vi "InitModuleManager.vi"(8 "error in (no error)":errorcluster, 10 "mmanager":path, 11 "SensorInfos":T6) -> (0 "error out (no error)":errorcluster, 3 "Sensor Engine Datas":T1[](array[typedef]) {"MM Frames"."payload" format="%x"; "MM Frames"."timestamp" format="%<%.7X\n%x>T"; "MM Frames"."type" items=["FlexRay Data"=32, "FlexRay Null"=33, "FlexRay Symbol"=34, "Log Trigger"=225, "Start Trigger"=226]; "MM Frames"."cycle count" max=63 step=1})   [LabVIEW 2023, in "MM.lvlib"]
uses:
  MM.lvlib
  Shared/SensorInfos.ctl
  Shared/SensorInfo.ctl
  Shared/Sensor Name.ctl
  Shared/Protocol.ctl
  MM Data.ctl
  MM Objects.ctl
  MM Object.ctl
  Sensor Engine Data.ctl
  <vilib>/xnet/xnet.llb/XNET Frame FlexRay.ctl
  <vilib>/xnet/xnet.llb/XNET Frame Type FlexRay.ctl
  <vilib>/xnet/xnet.llb/XNET String To IO Name (Signal).vi
  <vilib>/xnet/xnet.llb/XNET Create Session (Conversion).vi
  <resource>/objmgr/xnet.rc
  Shared/Vires VTD Shared.lvlib
  Engine/Vires VTD Engine.lvlib
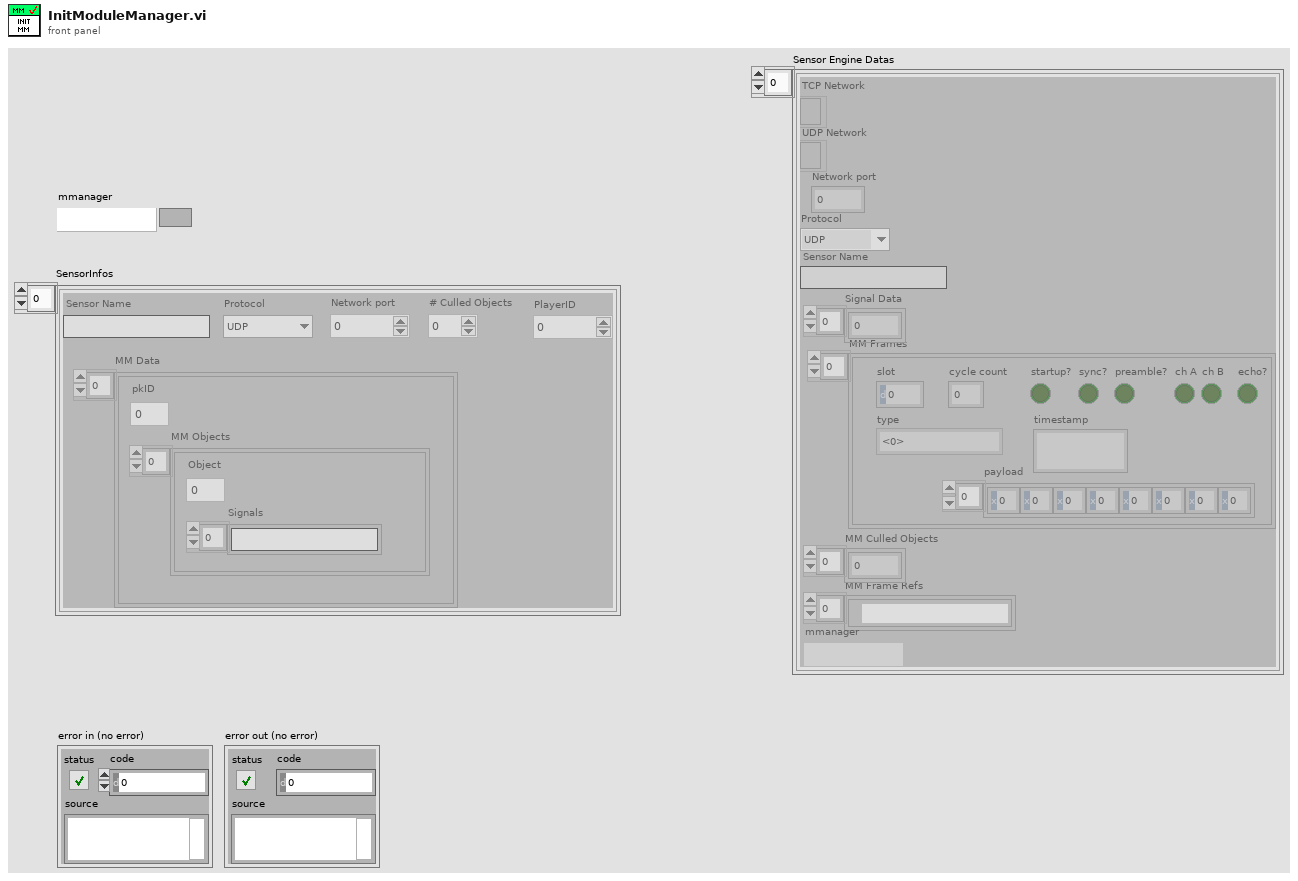
[diagram p1: front panel]
types:
  T1 = typedef "MM.lvlib/Sensor Engine Data.ctl" = cluster{"TCP Network":refnum<k5>, "UDP Network":refnum<k16>, "Network port":i32, "Protocol":T2, "Sensor Name":T3, "Signal Data":dbl[], "MM Frames":T4[], "MM Culled Objects":i32[], "MM Frame Refs":refnum<k21>[], "mmanager":path}
  T2 = typedef "Vires VTD Shared.lvlib/Protocol.ctl" = enum16{"UDP", "TCP"}
  T3 = typedef "Vires VTD Shared.lvlib/Sensor Name.ctl" = string
  T4 = typedef "XNET Frame FlexRay.ctl" = cluster{"timestamp":timestamp, "payload":u8[], "slot":u16, "type":T5, "cycle count":u8, "startup?":bool, "sync?":bool, "preamble?":bool, "ch A":bool, "ch B":bool, "echo?":bool}
  T5 = typedef "XNET Frame Type FlexRay.ctl" = u8
  T6 = typedef "Vires VTD Shared.lvlib/SensorInfos.ctl" = T7[]
  T7 = typedef "Vires VTD Shared.lvlib/SensorInfo.ctl" = cluster{"Sensor Name":T3, "Protocol":T2, "Network port":i32, "# Culled Objects":i32, "PlayerID":u8, "MM Data":T8}
  T8 = typedef "Vires VTD Shared.lvlib/MM Data.ctl" = T9[]
  T9 = typedef "MM.lvlib/MM Objects.ctl" = cluster{"pkID":i32, "MM Objects":T10[]}
  T10 = typedef "MM.lvlib/MM Object.ctl" = cluster{"Object":i32, "Signals":string[]}
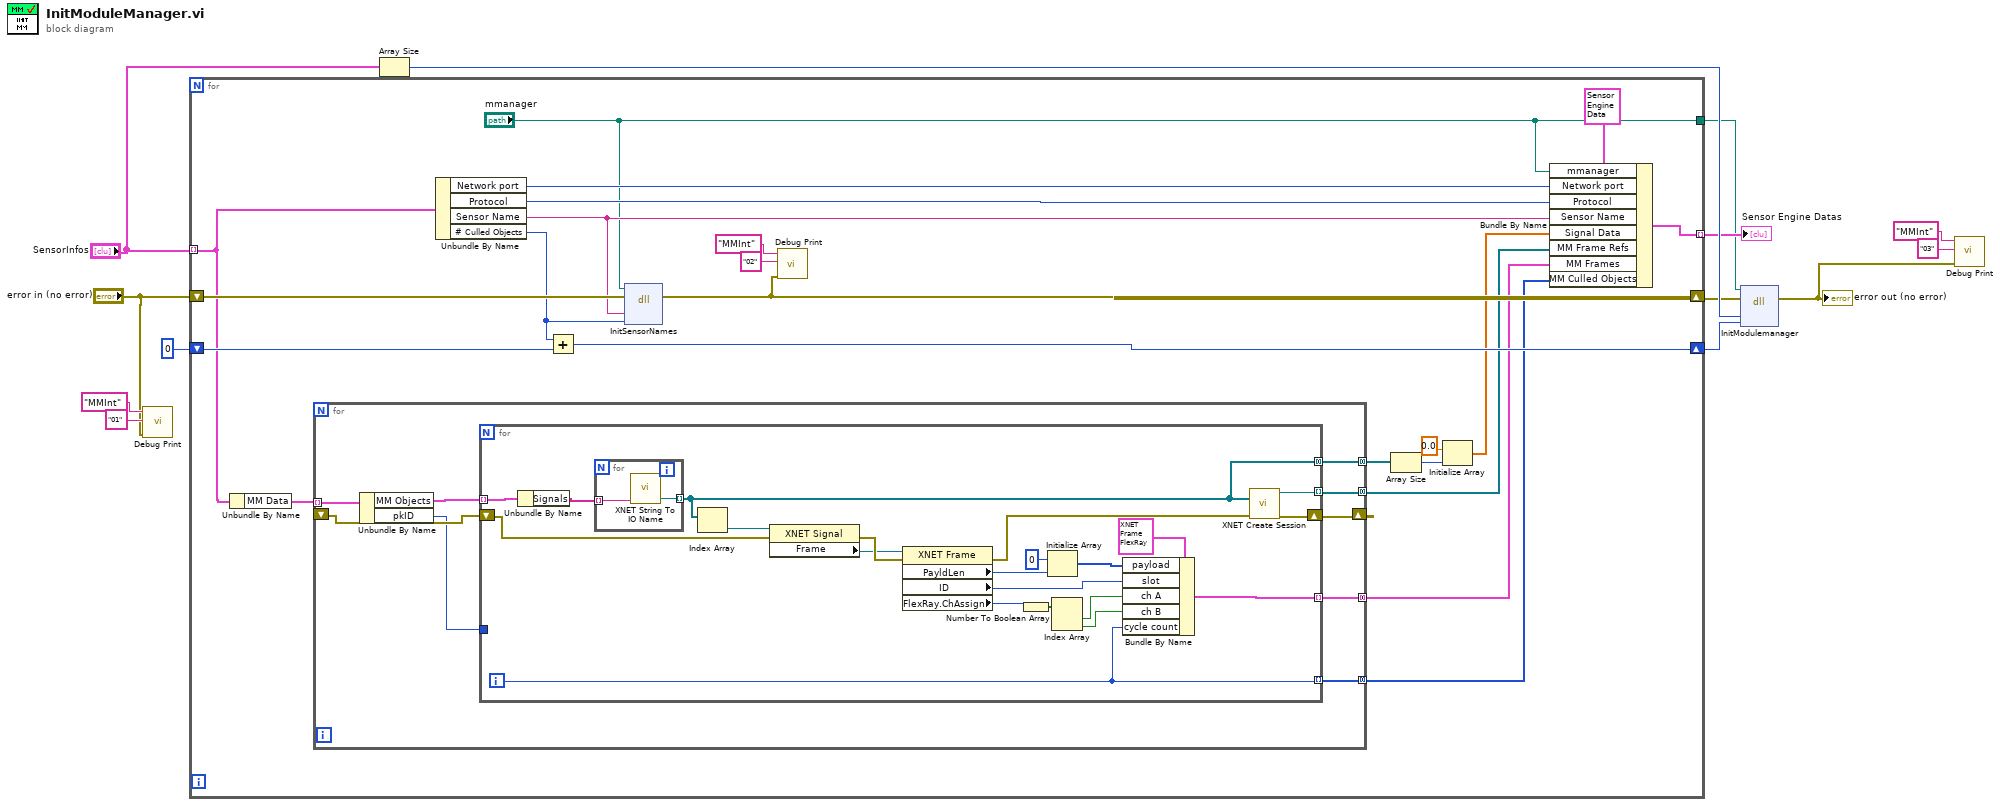
[diagram p0: block diagram]
diagram:
  n1 = call "Debug Print.vi"("error out"="error in (no error)", "Index"="01", "Module"="MMInt") -> ()  [unwired: 9 in]
  n2 = for {
    tunnel: "SensorInfos" -> [w31] mode=indexing
    shift-right: [w35] -> w11
    shift-left: 0 -> [w34]
    shift-right: [w14] -> w10
    shift-left: "error in (no error)" -> [w33]
    tunnel: [w19] -> w8 mode=indexing
    tunnel: ["mmanager"] -> w7
    n3 = Unbundle By Name(w31) -> ("MM Data"=w30:T8)
    n4 = for {
      shift-right: [w44] -> _
      shift-left: _ -> [w43]
      tunnel: [w42] -> w22 mode=concatenating
      tunnel: [w41] -> w21 mode=concatenating
      tunnel: w30 -> [w40] mode=indexing
      tunnel: [w37] -> w20 mode=concatenating
      tunnel: [w36] -> w18 mode=concatenating
      n5 = Unbundle By Name(w40) -> ("MM Objects"=w39:T10[], "pkID"=w38:i32)
      n6 = for {
        tunnel: [w52] -> w41 mode=indexing
        tunnel: [w48] -> w42 mode=indexing
        shift-right: [w50] -> w44
        shift-left: w43 -> [w49]
        tunnel: w39 -> [w47] mode=indexing
        tunnel: w38 -> [_]
        tunnel: [w46] -> w37 mode=indexing
        tunnel: [w45] -> w36 mode=concatenating
        i -> [w46]
        n7 = Unbundle By Name(w47) -> ("Signals"=w65:string[])
        n8 = for {
          tunnel: w65 -> [w67] mode=indexing
          tunnel: [w66] -> w45 mode=indexing
          n9 = call-poly <vilib>:"XNET String To IO Name.vi"("string"=w67) -> ("XNET Signal"=w66:refnum<k21>)  [unwired: 4 out]
        }
        n10 = Index Array(array=w45) -> (element=w53:refnum<k21>)  [unwired: 1 in]
        n11 = property class="XNET Signal"(reference=w53, error in=w49) -> (error out=w64:errorcluster, "Frame"=w63:refnum<k21>)  [unwired: 1 out]
        n12 = property class="XNET Frame"(reference=w63, error in=w64) -> (error out=w51:errorcluster, "PayldLen"=w56:u32, "ID"=w58:u32, "FlexRay.ChAssign"=w59:u32)  [unwired: 1 out]
        n13 = Number To Boolean Array(number=w59) -> (Boolean array=w54:bool[])
        n14 = Initialize Array(u8 0 ("element"), w56) -> (w57:u8[])
        n15 = Index Array(array=w54) -> (element #1=w60:bool, element #2=w61:bool)  [unwired: 2 in]
        n16 = Bundle By Name(cluster=T4 {"timestamp"=timestamp(0 s since 1904-01-01), "payload"=[], "slot"=1, "type"=32, "cycle count"=0, "startup?"=FALSE, "sync?"=FALSE, "preamble?"=FALSE, "ch A"=FALSE, "ch B"=FALSE, "echo?"=FALSE} ("FlexRay frame"), "payload"=w57, "slot"=w58, "ch A"=w60, "ch B"=w61, "cycle count"=w46) -> (w52:T4)
        n17 = call-poly <vilib>:"XNET Create Session.vi"("signal list"=w45, "error in (no error)"=w51) -> ("session out"=w48:refnum<k21>, "error out"=w50:errorcluster)  [unwired: 12 in]
      }
    }
    n18 = Unbundle By Name(w31) -> ("Network port"=w26:i32, "Protocol"=w25:T2, "Sensor Name"=w24:T3, "# Culled Objects"=w32:i32)
    n19 = Add(x=w32, y=w34) -> (x+y=w35:i32)
    n20 = dll-call lib="ModuleManager.dll" fn="InitSensorNames"(path in="mmanager", error in=w33, "SensorName"=w24, "noCulledObj"=w32) -> (error out=w14:errorcluster)  [unwired: 4 in, 1 out]
    n21 = call "Debug Print.vi"("error out"=w14, "Index"="02", "Module"="MMInt") -> ()  [unwired: 9 in]
    n22 = Array Size(array=w18) -> (size(s)=w28:i32)
    n23 = Initialize Array(0.0, w28) -> (w23:dbl[])
    n24 = Bundle By Name(cluster=T1 {"TCP Network"=refnum, "UDP Network"=refnum, "Network port"=0, "Protocol"=enum."UDP", "Sensor Name"="", "Signal Data"=[], "MM Frames"=[], "MM Culled Objects"=[], "MM Frame Refs"=[], "mmanager"=path ""} ("MM.lvlib:Sensor Engine Data"), "mmanager"="mmanager", "Network port"=w26, "Protocol"=w25, "Sensor Name"=w24, "Signal Data"=w23, "MM Frame Refs"=w22, "MM Frames"=w21, "MM Culled Objects"=w20) -> (w19:T1)
  }
  "Sensor Engine Datas" <- w8
  n25 = Array Size(array="SensorInfos") -> (size(s)=w12:i32)
  n26 = dll-call lib="ModuleManager.dll" fn="InitModulemanager"(path in=w7, error in=w10, "noSensor"=w12, "noCulledObj"=w11) -> (error out=w1:errorcluster)  [unwired: 4 in, 1 out]
  "error out (no error)" <- w1
  n27 = call "Debug Print.vi"("error out"=w1, "Index"="03", "Module"="MMInt") -> ()  [unwired: 9 in]
